vi "Exemple_Metrics_Calinski_Harabasz_Score.vi"() -> ()   [LabVIEW 2020]
uses:
  Objet/3 - Model selection and evaluation/3.3 - Metrics and scoring/calinski_harabasz_score/Calinski_Harabasz_Score.vi
panel:
  out "Score":string
  out "error out":errorcluster caption="sortie d'erreur"
  in  "error in (no error)":errorcluster caption="entrée d'erreur (pas d'erreur)"
  in  "labels":string[][](array[string])=[["1"], ["1"], ["0"], ["0"]]
  in  "X":string[][](array[string])=[["5,1", "3,5", "1,4", "0,2"], ["4,9", "3", "1,4", "0,2"], ["4,7", "3,2", "1,3", "0,2"], ["4,6", "3,1", "1,5", "0,2"]]
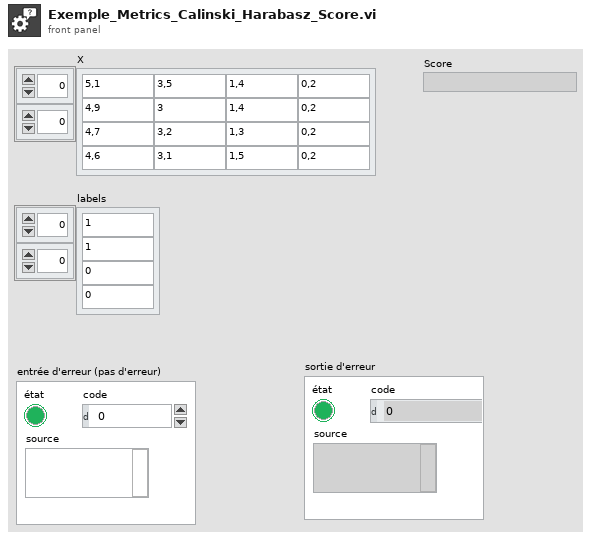
[diagram p1: front panel]
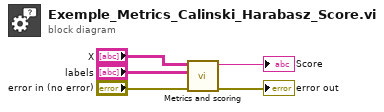
[diagram p0: block diagram]
diagram:
  n1 = call-poly "Metrics and scoring.vi"("error in (no error)"="error in (no error)", "labels"="labels", "X"="X") -> ("error out"=→"error out":errorcluster, "Score"=→"Score":string)  [unwired: 7 in]
